vi "CoPilot Analyze.vi"(0 "JoystickDevRef":T1, 2 "Extra throttle":dbl) -> (1 "ConveyerBelt":dbl, 8 "Shoot Motors":dbl, 15 "La Fire at will?":bool)   [LabVIEW 2012]
uses:
  <vilib>/Rock Robotics/WPI/Joystick/WPI_JoystickDevRef.ctl
  <vilib>/Rock Robotics/WPI/Joystick/WPI_JoystickDeviceEnum.ctl
  BotStatus.vi
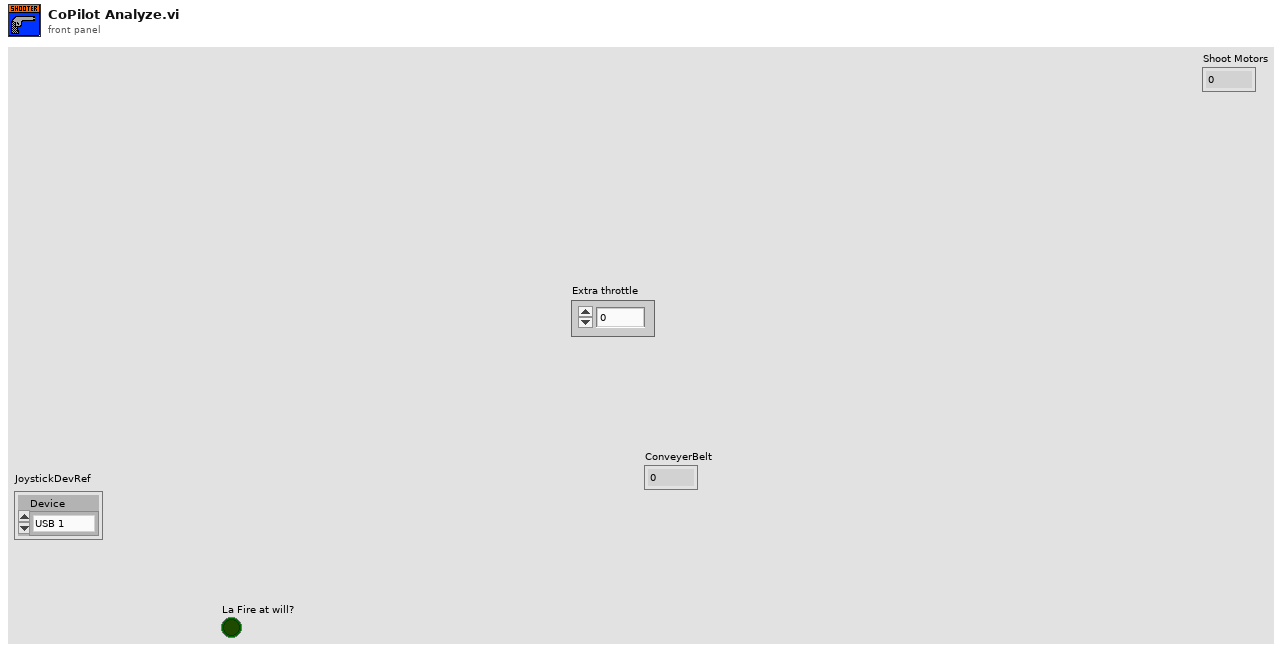
[diagram p1: front panel]
types:
  T1 = typedef "WPI_JoystickDevRef.ctl" = cluster{"Device":T2}
  T2 = typedef "WPI_JoystickDeviceEnum.ctl" = enum16{"USB 1", "USB 2", "USB 3", "USB 4", "Kinect 1", "Kinect 2"}
  T3 = typedef "WPI_JoystickButtonState.ctl" = cluster{"Button 1":bool, "Button 2":bool, "Button 3":bool, "Button 4":bool, "Button 5":bool, "Button 6":bool, "Button 7":bool, "Button 8":bool, "Button 9":bool, "Button 10":bool, "Button 11":bool, "Button 12":bool}
  T4 = cluster{"axis 1 (x)":dbl, "axis 2 (y)":dbl, "axis 3 (throttle)":dbl, "axis 4":dbl, "axis 5":dbl, "axis 6":dbl}
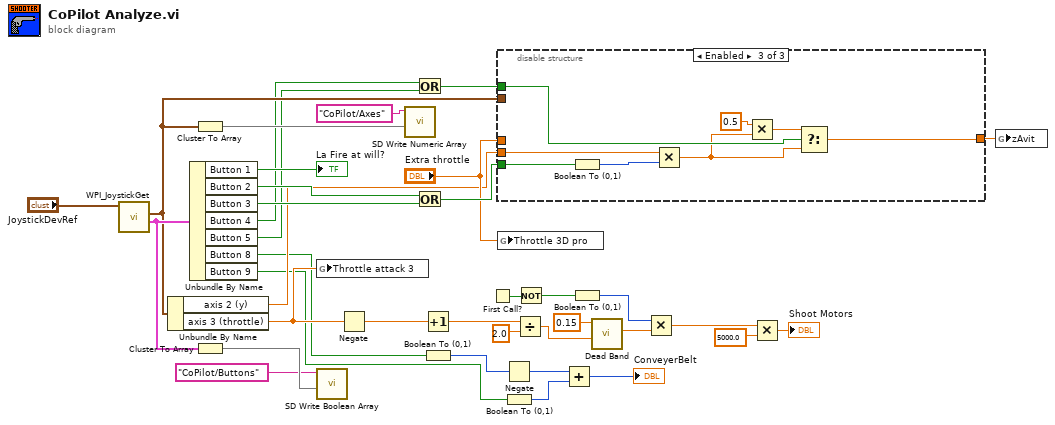
[diagram p0: block diagram]
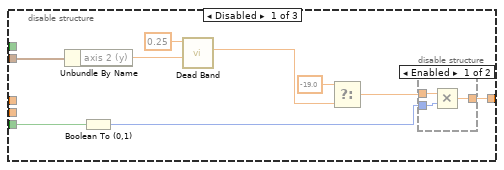
[diagram p2: hidden frame]
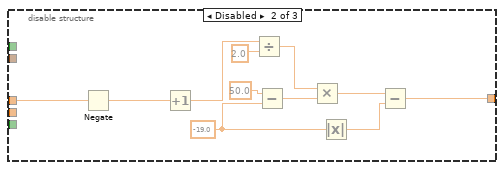
[diagram p4: hidden frame]
diagram:
  n1 = call <vilib>:"WPI_JoystickGet.vi"("JoystickDevRef"="JoystickDevRef") -> ("Buttons"=w28:T3, "Axes"=w12:T4)  [unwired: 4 in, 1 out]
  n2 = Unbundle By Name(w12) -> ("axis 2 (y)"=w7:dbl, "axis 3 (throttle)"=w9:dbl)
  n3 = Unbundle By Name(w28) -> ("Button 1"=→"La Fire at will?":bool, "Button 2"=w30:bool, "Button 3"=w29:bool, "Button 4"=w3:bool, "Button 5"=w2:bool, "Button 8"=w4:bool, "Button 9"=w5:bool)
  n4 = Cluster To Array(cluster=w12) -> (array=w33:dbl[])
  n5 = Cluster To Array(cluster=w28) -> (array=w35:bool[])
  n6 = global write "BotStatus.vi" "Throttle attack 3"(w9) -> ()
  n7 = call <vilib>:"SD Write Boolean Array.vi"("Boolean Array"=w35, "Name"="CoPilot/Buttons") -> ()  [unwired: 8 in, 2 out]
  n8 = Negate(x=w9) -> (-x=w18:dbl)
  n9 = call <vilib>:"SD Write Numeric Array.vi"("Numeric Array"=w33, "Name"="CoPilot/Axes") -> ()  [unwired: 8 in, 2 out]
  n10 = Or(x=w3, y=w2) -> (x .or. y?=w1:bool)
  n11 = Or(x=w30, y=w29) -> (x .or. y?=w27:bool)
  n12 = Increment(x=w18) -> (x+1=w20:dbl)
  n13 = Boolean To (0,1)(Boolean=w4) -> (0, 1=w26:i16)
  n14 = First Call?() -> (First Call?: T/F=w23:bool)
  n15 = disable-structure shown="Enabled" {
    disable-tunnel: [w45 w50 w64] -> w11
    disable-tunnel: w27 -> [w44 _ w68]
    disable-tunnel: w12 -> [w39 _ _]
    disable-tunnel: "Extra throttle" -> [_ w57 _]
    disable-tunnel: w7 -> [_ _ w66]
    disable-tunnel: w1 -> [_ _ w65]
    frame Disabled {
      n16 = Unbundle By Name(w39) -> ("axis 2 (y)"=w41:dbl)
      n17 = Boolean To (0,1)(Boolean=w44) -> (0, 1=w43:i16)
      n18 = call "Dead Band.vi"("Axis In"=w41, "Dead Band"=0.25) -> ("Axis Out"=w42:dbl)  [unwired: 9 in]
      n19 = Select(t=-19.0, f=w42) -> (s? t:f=w40:dbl)  [unwired: 1 in]
      n20 = disable-structure shown="Enabled" {
        disable-tunnel: w40 -> [w48 w49]
        disable-tunnel: [w47 w49] -> w45
        disable-tunnel: w43 -> [w46 _]
        frame Enabled {
          n21 = Multiply(x=w48, y=w46) -> (x*y=w47:dbl)
        }
        frame Disabled {
        }
      }
    }
    frame Disabled {
      w52 = -19.0 ("y")
      n22 = Negate(x=w57) -> (-x=w60:dbl)
      n23 = Increment(x=w60) -> (x+1=w58:dbl)
      n24 = Divide(x=w58, y=2.0) -> (x/y=w56:dbl)
      n25 = Subtract(x=50.0 ("y"), y=w52) -> (x-y=w54:dbl)
      n26 = Multiply(x=w56, y=w54) -> (x*y=w53:dbl)
      n27 = Absolute Value(x=w52) -> (abs(x)=w51:dbl)
      n28 = Subtract(x=w53, y=w51) -> (x-y=w50:dbl)
    }
    frame Enabled {
      n29 = Boolean To (0,1)(Boolean=w68) -> (0, 1=w67:i16)
      n30 = Multiply(x=w66, y=w67) -> (x*y=w62:dbl)
      n31 = Multiply(x=0.5, y=w62) -> (x*y=w63:dbl)
      n32 = Select(t=w63, s=w65, f=w62) -> (s? t:f=w64:dbl)
    }
  }
  n33 = global write "BotStatus.vi" "Throttle 3D pro"("Extra throttle") -> ()
  n34 = Negate(x=w26) -> (-x=w25:i16)
  n35 = Boolean To (0,1)(Boolean=w5) -> (0, 1=w24:i16)
  n36 = Divide(x=w20, y=2.0) -> (x/y=w15:dbl)
  n37 = Not(x=w23) -> (.not. x?=w22:bool)
  n38 = Add(x=w25, y=w24) -> (x+y=→"ConveyerBelt":i16)
  n39 = Boolean To (0,1)(Boolean=w22) -> (0, 1=w21:i16)
  n40 = call "Dead Band.vi"("Axis In"=w15, "Dead Band"=0.15) -> ("Axis Out"=w13:dbl)  [unwired: 9 in]
  n41 = Multiply(x=w21, y=w13) -> (x*y=w14:dbl)
  n42 = Multiply(x=w14, y=5000.0 ("Dead Band")) -> (x*y=→"Shoot Motors":dbl)
  n43 = global write "BotStatus.vi" "zAvit"(w11) -> ()
